vi "DataReader.vi"(11 "Filename":path=path "D:/Sonify Labview/Data/PorkSkin_40C_5Min.lvm") -> ()   [LabVIEW 2015]
panel:
  out "error out":errorcluster
  out "Acoustic Pressure":dbl[](graph) caption="Signals"
  out "Thermal Dose (Min)":dbl format="%#_2g"
  out "Drive Voltage":dynamicdata(graph) caption="Signals"
  out "Temperature":dynamicdata(graph) caption="Signals"
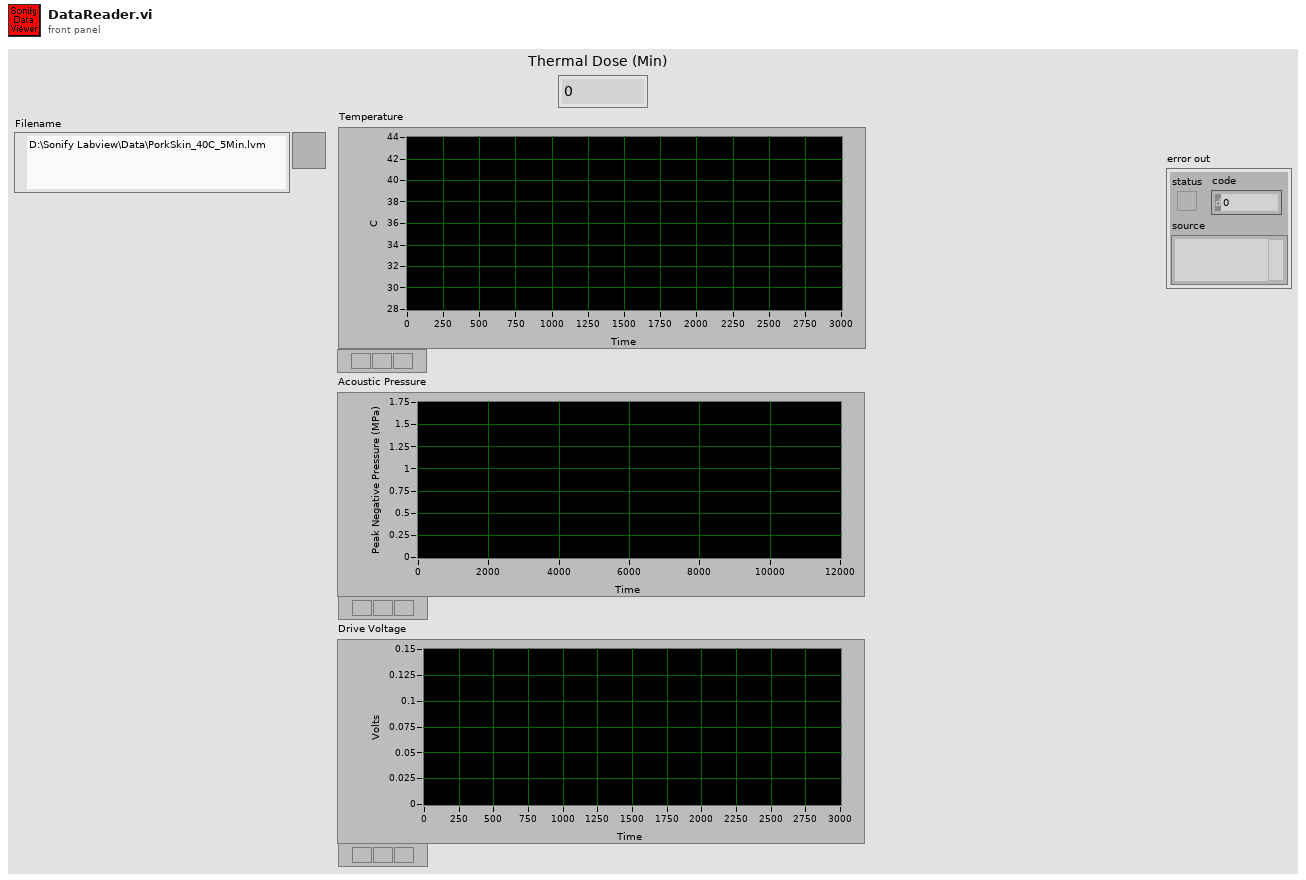
[diagram p1: front panel]
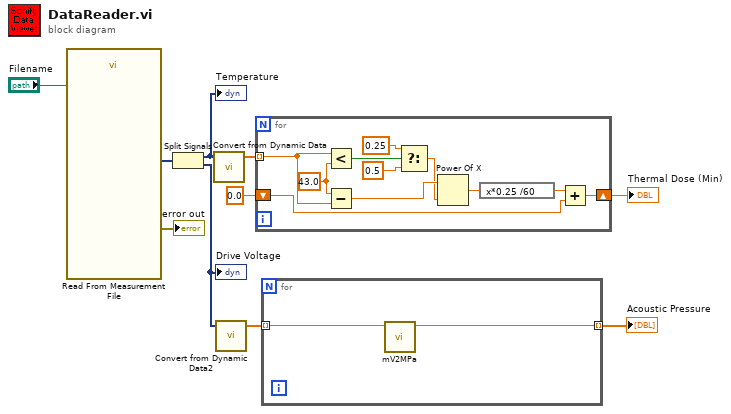
[diagram p0: block diagram]
diagram:
  n1 = call "Read From Measurement File"("Filename"="Filename") -> ("error out"=→"error out":errorcluster, "Signals"=w10:dynamicdata)  [unwired: 5 in, 4 out]
  n2 = Split Signals(w10) -> (w8:dynamicdata, w4:dynamicdata)  [unwired: 2 in]
  "Temperature" <- w8
  "Drive Voltage" <- w4
  n3 = call "Convert from Dynamic Data"("Dynamic Data Type"=w8) -> ("Array"=w7:dbl[])  [unwired: 3 in]
  n4 = call "Convert from Dynamic Data2"("Dynamic Data Type"=w4) -> ("Array"=w2:dbl[])  [unwired: 3 in]
  n5 = for {
    tunnel: w7 -> [w18] mode=indexing
    shift-right: [w15] -> w5
    shift-left: 0.0 -> [w14]
    w11 = 43.0 ("y")
    n6 = Less?(x=w18, y=w11) -> (x < y?=w21:bool)
    n7 = Subtract(x=w11, y=w18) -> (x-y=w13:dbl)
    n8 = Select(t=0.25, s=w21, f=0.5) -> (s? t:f=w12:dbl)
    n9 = Power Of X(1:w12, 2:w13) -> (0:w17:dbl)
    n10 = expression code="x*0.25 /60"(w17) -> (w16:dbl)
    n11 = Add(x=w16, y=w14) -> (x+y=w15:dbl)
  }
  "Thermal Dose (Min)" <- w5
  n12 = for {
    tunnel: [w22] -> w3 mode=indexing
    tunnel: w2 -> [w23] mode=indexing
    n13 = call "mV2MPa.vi"("Volts In"=w23) -> ("MPa Out"=w22:dbl)  [unwired: 10 in]
  }
  "Acoustic Pressure" <- w3
